vi "Set Jerk Rate.vi"(4 "error in (no error)":errorcluster, 5 "Vector Jerk (0 units/s^3)":dbl min=0.0 max=2000000000.0 format="%.4g", 6 "Axis (1)":i32=1 min=1 max=3, 7 "VISA resource name":refnum<visa-resource-name>) -> (0 "error out":errorcluster, 3 "VISA resource name out":refnum<visa-resource-name>)   [LabVIEW 2012, in "Newport ESP301.lvlib"]
doc: "This command is used to set the jerk (i.e., rate of change in acceleration) value for an axis. Its execution is immediate, meaning that the jerk is altered when the command is processed and trajectory mode is set to S-curve, even while a motion is in progress. It can be used as an immediate command or inside a program.\nNote:\nAvoid changing the jerk during the acceleration or deceleration periods.\nFor better predictable results, change jerk only when the axis is not\nmoving."
uses:
  Newport ESP301.lvlib
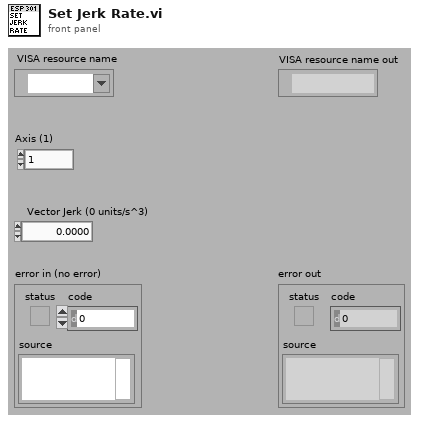
[diagram p1: front panel]
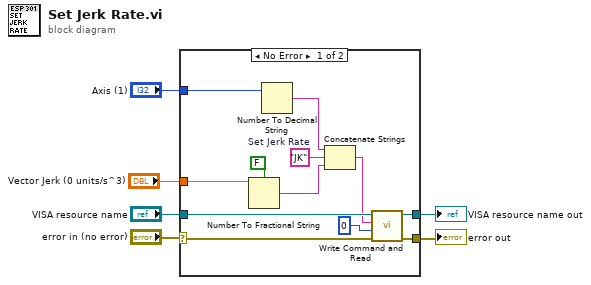
[diagram p0: block diagram]
diagram:
  n1 = case shown="No Error" "error in (no error)" {
    selector: "error in (no error)" -> [w15 w20]
    tunnel: [w17 w20] -> w6
    tunnel: "VISA resource name" -> [w18 w19]
    tunnel: [w16 w19] -> w5
    tunnel: "Axis (1)" -> [w11 _]
    tunnel: "Vector Jerk (0 units/s^3)" -> [w8 _]
    frame No Error {
      w14 = "JK"  # Set Jerk Rate
      n2 = Number To Fractional String(use system decimal point (T)=FALSE ("utiliser le séparateur décimal du système (V)"), number=w8) -> (F-format string=w9:string)  [unwired: 2 out]
      n3 = Number To Decimal String(number=w11) -> (decimal integer string=w13:string)  [unwired: 1 in]
      n4 = Concatenate Strings(w13, w14, w9) -> (w12:string)
      n5 = call "Write Command and Read.vi"("error in (no error)"=w15, "Bytes to read (100)"=u32 0, "Command"=w12, "VISA resource name"=w18) -> ("error out"=w17:errorcluster, "VISA resource name out"=w16:refnum<visa-resource-name>)  [unwired: 3 in, 1 out]
    }
    frame Error {
    }
  }
  "error out" <- w6
  "VISA resource name out" <- w5
